vi "10V_Bits.vi"(11 "Numeric":dbl) -> (3 "Bits":string)   [LabVIEW 2015]
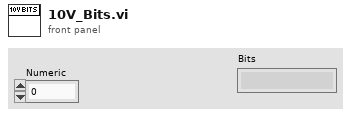
[diagram p1: front panel]
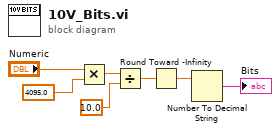
[diagram p0: block diagram]
diagram:
  n1 = Multiply(x="Numeric", y=4095.0) -> (x*y=w5:dbl)
  n2 = Divide(x=w5, y=10.0) -> (x/y=w3:dbl)
  n3 = Round Toward -Infinity(1:w3) -> (0:w2:dbl)
  n4 = Number To Decimal String(number=w2) -> (decimal integer string=→"Bits":string)  [unwired: 1 in]
